vi "ZLIB Deflate__ogtk.vi"(4 "error in (no error)":errorcluster, 6 "compression level (default)":i32=-1, 7 "input":string) -> (0 "error out":errorcluster, 2 "length":i32, 3 "deflated output":string)   [LabVIEW 2020]
doc: "Compresses data passed into \"input\". Valid compressions levels are 0(least) to 9(greatest) with 0 being no compression. Compression level -1 is the default compression for the zlib library and is normally equal to 6. Returns the deflated output data, and the length of the output.\n\nReturns \"Generic Error\" (42) when the zlib routine encountered any errors."
uses:
  <userlib>/_OpenG.lib/lvzip/lvzlib.dll
panel:
  # "`"
  # "Please visit http://www.OpenG.org to learn about the\nOpen Source LabVIEW software movement.\n\nNOTICE -- YOU MUST LEAVE THIS NOTICE IN PLACE.  PER THE TERMS OF THE LICENSE BELOW, YOU MAY SUBLICENSE THIS SOFTWARE \nIN ANY WAY THAT DOES NOT CONFLICT WITH THIS LICENSE.\n\n### BSD License (http://www.opensource.org/licenses/bsd-license.php) Begin ###\n \nCopyright (C) 2002 Rolf Kalbermatter rolf.kalbermatter@citeng.com\n\nAll rights reserved.\n\nRedistribution and use in source and binary forms, with or without modification, are permitted provided that the following conditions are met:\n\n    * Redistributions of source code must retain the above copyright notice, this list of conditions and the following disclaimer.\n    * Redistributions in binary form must reproduce the above copyright notice, this list of conditions and the following disclaimer in the \n       documentation and/or other materials provided with the distribution.\n    * Neither the name of SciWare, James Kring, Inc., nor the names of its contributors may be used to endorse or promote products derived \n       from this software without specific prior written permission.\n\nTHIS SOFTWARE IS PROVIDED BY THE COPYRIGHT HOLDERS AND CONTRIBUTORS \"AS IS\" AND ANY EXPRESS OR IMPLIED WARRANTIES, \nINCLUDING, BUT NOT LIMITED TO, THE IMPLIED WARRANTIES OF MERCHANTABILITY AND FITNESS FOR A PARTICULAR PURPOSE ARE \nDISCLAIMED. IN NO EVENT SHALL THE COPYRIGHT OWNER OR CONTRIBUTORS BE LIABLE FOR ANY DIRECT, INDIRECT, INCIDENTAL,\n SPECIAL, EXEMPLARY, OR CONSEQUENTIAL DAMAGES (INCLUDING, BUT NOT LIMITED TO, PROCUREMENT OF SUBSTITUTE GOODS OR \nSERVICES; LOSS OF USE, DATA, OR PROFITS; OR BUSINESS INTERRUPTION) HOWEVER CAUSED AND ON ANY THEORY OF LIABILITY, \nWHETHER IN CONTRACT, STRICT LIABILITY, OR TORT (INCLUDING NEGLIGENCE OR OTHERWISE) ARISING IN ANY WAY OUT OF THE USE \nOF THIS SOFTWARE, EVEN IF ADVISED OF THE POSSIBILITY OF SUCH DAMAGE.\n\n### BSD License End ###"
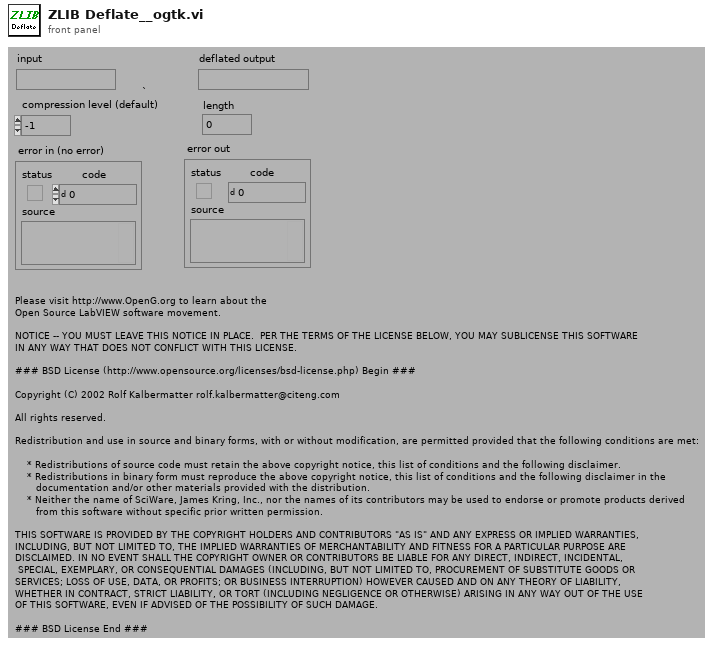
[diagram p1: front panel]
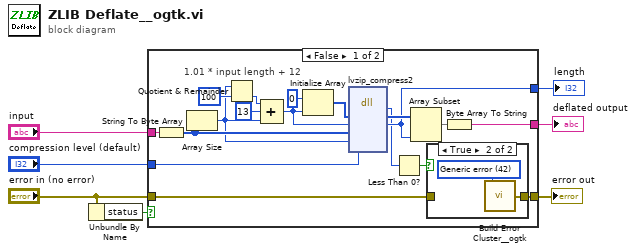
[diagram p0: block diagram]
diagram:
  n1 = Unbundle By Name("error in (no error)") -> ("status"=w7:bool)
  n2 = case shown="False" w7 {
    tunnel: "error in (no error)" -> [w24 w31]
    tunnel: [w23 w31] -> w5
    tunnel: [w12 "" ("string")] -> w4
    tunnel: [w11 0 ("destLen")] -> w3
    tunnel: "input" -> [w10 _]
    tunnel: "compression level (default)" -> [w9 _]
    frame False {
      # "1.01 * input length + 12"
      n3 = String To Byte Array(string=w10) -> (unsigned byte array=w22:u8[])
      n4 = Array Size(array=w22) -> (size(s)=w15:i32)
      n5 = Quotient & Remainder(x=w15, y=100) -> (floor(x/y)=w18:i32)  [unwired: 1 out]
      n6 = Compound Arithmetic op=ADD(w18, 13 ("x"), w15) -> (w20:i32)
      n7 = Initialize Array(u8 0, w20) -> (w21:u8[])
      n8 = dll-call lib="C:/Work/OpenG/opengtoolkit/lvzip/source/lvzlib.*" fn="lvzip_compress2"("pDest"=w21, "destLen"=w20, "pSource"=w22, "sourceLen"=w15, "level"=w9) -> (w8:i32, "pDest"=w14:u8[], "destLen"=w11:i32)  [unwired: 6 in, 2 out]
      n9 = Less Than 0?(x=w8) -> (x < 0?=w25:bool)
      n10 = Array Subset(array=w14, length=w11) -> (w13:u8[])  [unwired: 1 in]
      n11 = case shown="True" w25 {
        tunnel: [w26 w28] -> w23
        tunnel: w24 -> [w26 _]
        frame False {
        }
        frame True {
          w27 = 42 items=["No error", "Argument error", "Memory is full", "Out of zone", "End of file", "File already open", "Generic file I/O error", "File not found", "File permission error", "Disk is full", "Duplicate path", "Too many files open", "System feature not enabled", "Resource file not found", "Cannot add resource", "Resource not found", "Image not found", "Image memory error", "Pen does not exist", "Config type invalid", "Config token not found", "Config parse error", "Config memory error", "Bad external code format", "Bad external code offset", "External code not present", "Null window", "Destroy window error", "Null menu", "Print aborted", "Bad print record", "Print driver error", "Windows error during printing", "Memory error during printing", "Print dialog error", "Generic print error", "Invalid device refnum", "Device not found", "Device parameter error", "Device unit error", "Cannot open device", "Device call aborted", "Generic error", "Cancelled by user", "Object ID too low", "Object ID too high", "Object not in heap", "Unknown heap", "Unknown object (invalid DefProc)", "Unknown object (DefProc not in table)", "Message out of range", "Invalid (null) method", "Unknown message", "Manager call not supported", "Bad address", "Network operation in progress", "Network operation timed out", "Connection is busy", "Network attribute not supported", "Network error", "Address in use", "System out of memory", "Connection aborted", "Connection refused", "Not connected", "Already connected", "Connection closed", "Initialization error (interapplication manager)", "Bad occurrence", "Wait on unbound occurrence handler", "Occurrence queue overflow", "Datalog type conflict", "Unused", "Unrecognized type (interapplication manager)", "Memory corrupt", "Failed to make temporary DLL", "Old CIN version", "Drag socket not found", "Failed to load drop-object", "Failed to register OLE object", "Failed to release OLE object", "Format specifier type mismatch", "Unknown format specifier", "Too few format specifiers", "Too many format specifiers", "Scan failed", "Newer CIN version", "Error converting to variant", "Runtime menu error", "Password tampered", "Variant attribute not found", "Incompatible variant data type", "Event data is not available", "Event Store is not present", "Occurrence is not found", "Event Queue is not created", "Event info is not available", "Refnum passed is NULL", "Error retrieving Class GUID", "Error retrieving CoClass GUID", "Error retrieving TypeLib GUID.", "Bad built application magic bytes.", "Specific driver is different from the specific driver associated with the Logical Name.", "There is no session opened to the class driver.", "Max Error", "MAX - Error with config objects", "MAX - Error loading configuration", "MAX - Group not supported"]
          n12 = call <userlib>:"Build Error Cluster__ogtk.vi"("code"=w27) -> ("error out"=w28:errorcluster)  [unwired: 1 in]
        }
      }
      n13 = Byte Array To String(unsigned byte array=w13) -> (string=w12:string)
    }
    frame True {
    }
  }
  "error out" <- w5
  "deflated output" <- w4
  "length" <- w3
